vi "Parse multiple measurements to display - DLTS.vi"(0 "Array":T1[](array[typedef]) {"DLTS properties"."V range" items=["10mV"=0.01, "100mV"=0.1, "1V"=1.0, "10V"=10.0]; "DLTS properties"."I range" items=["10mV"=0.01, "100mV"=0.1, "1V"=1.0, "10V"=10.0]}, 5 "Session properties":T3, 7 "Workspace":path, 9 "Loop data":T4={"Persistent"={"Last file"=path "", "Last user"="", "Users"=[]}, "Temp handle"={"Connected"=FALSE, "Temp ctrl"={"Gain (P)"=0.0, "Reset (I)"=0.0, "Rate (D)"=0.0, "Stabilization rate"=0.0, "Stabilization delta"=0.0, "Type"=enum."Lake Shore 325", "Custom temp ctrl"={"VISA resource name"=""}, "Lakeshore 325"={"VISA name"="", "Loop"=0, "Heater Range"=1, "Heater Resistance"=0, "Sample sensor"=0, "Fast sensor"=0, "Slow sensor"=0}, "Lakeshore 331"={"VISA name"="", "Loop"=1, "Heater Range"=0, "Sample sensor"=0, "Fast sensor"=0, "Slow sensor"=0}, "Lakeshore 332"={"VISA name"="", "Loop"=1, "Heater Range"=0, "Sample sensor"=0, "Fast sensor"=0, "Slow sensor"=0}, "Lakeshore 335"={"VISA name"="", "Loop"=1, "Sample sensor"=0, "Fast sensor"=0, "Slow sensor"=0}}}, "Paths"={"Manual"=path "", "Settings"=path "", "Persistent"=path "", "Work dir."=path ""}, "Settings"={"MFIA"={"Address"="", "Use compensation"=TRUE, "Shut down gracefully"=FALSE}, "Temp ctrl"={"Gain (P)"=0.0, "Reset (I)"=0.0, "Rate (D)"=0.0, "Stabilization rate"=0.0, "Stabilization delta"=0.0, "Type"=enum."Lake Shore 325", "Custom temp ctrl"={"VISA resource name"=""}, "Lakeshore 325"={"VISA name"="", "Loop"=0, "Heater Range"=1, "Heater Resistance"=0, "Sample sensor"=0, "Fast sensor"=0, "Slow sensor"=0}, "Lakeshore 331"={"VISA name"="", "Loop"=1, "Heater Range"=0, "Sample sensor"=0, "Fast sensor"=0, "Slow sensor"=0}, "Lakeshore 332"={"VISA name"="", "Loop"=1, "Heater Range"=0, "Sample sensor"=0, "Fast sensor"=0, "Slow sensor"=0}, "Lakeshore 335"={"VISA name"="", "Loop"=1, "Sample sensor"=0, "Fast sensor"=0, "Slow sensor"=0}}, "Source-meter"={"Type"=enum."Custom", "Custom source-meter"={"VISA resource name"=""}, "Keithley 2600"={"VISA name"=""}}, "Other"={"Enable OriginLab"=FALSE, "Reader mode"=FALSE, "Auto-save"=FALSE}, "Defaults"={"IV properties"={"T"=0.0, "Vstart"=-0.5, "Vstop"=0.5, "Vpoints"=10.0, "Settling"=0.01, "I limit"=0.1, "Log mapping"=FALSE, "Averaging"=0.0}, "CV properties"={"T"=0.0, "Vstart"=-0.5, "Vstop"=0.5, "Vpoints"=10.0, "Precision"=enum."Normal", "Test signal"=0.01, "Auto I range"=FALSE, "Test frequency"=100000.0, "I range"=-2.0, "V range"=10.0, "Log mapping"=FALSE, "Rel perm"=0.0, "Area"=0.0}, "DLTS properties"={"Tstart"=0.0, "Instant start"=FALSE, "Tstop"=0.0, "T rate"=0.0, "Test signal"=0.0, "Test frequency"=0.0, "Bandwidth"=0.0, "Averaging"=0.0, "Vbias"=0.0, "Vpulse"=0.0, "pulse length"=0.0, "Pulse 2"=FALSE, "Vpulse 2"=0.0, "pulse length 2"=0.0, "I range"=-2.0, "V range"=10.0, "Emission rate"=[], "Sampling rate"=0.0, "Acq. delay"=0.0}, "LDLTS properties"={"T"=0.0, "Test signal"=0.0, "Test frequency"=0.0, "Bandwidth"=0.0, "Averaging"=0.0, "Vbias"=0.0, "Vpulse"=0.0, "pulse length"=0.0, "Pulse 2"=FALSE, "Vpulse 2"=0.0, "pulse length 2"=0.0, "I range"=-2.0, "V range"=10.0, "Sampling rate"=0.0, "Acq. delay"=0.0, "Sampling time"=0.0}}}, "Software version"=0.0, "MFIA handle"={"ziHandle"={"handleValid"=FALSE, "Conn"=0, "Path Prefix"="", "Handle"=0, "Connected"=FALSE, "Clockbase(s)"=0.0}, "Selected device"="", "ziModHandle"={"handleValid"=FALSE, "Conn"=0, "ModHandle"=0, "moduleID"="", "Path Prefix"=""}}, "Source-meter handle"={"Connected"=FALSE, "Source-meter"={"Type"=enum."Custom", "Custom source-meter"={"VISA resource name"=""}, "Keithley 2600"={"VISA name"=""}}}} {"MFIA handle"."ziModHandle"."ModHandle" format="0x%08x"; "MFIA handle"."ziModHandle"."Conn" format="0x%08x"; "MFIA handle"."ziHandle"."Handle" format="0x%08x"; "MFIA handle"."ziHandle"."Conn" format="0x%08x"; "Settings"."Defaults"."LDLTS properties"."V range" items=["10mV"=0.01, "100mV"=0.1, "1V"=1.0, "10V"=10.0]; "Settings"."Defaults"."LDLTS properties"."I range" items=["100nA"=-7.0, "1µA"=-6.0, "10µA"=-5.0, "100µA"=-4.0, "1mA"=-3.0, "10mA"=-2.0]; "Settings"."Defaults"."DLTS properties"."V range" items=["10mV"=0.01, "100mV"=0.1, "1V"=1.0, "10V"=10.0]; "Settings"."Defaults"."DLTS properties"."I range" items=["10mV"=0.01, "100mV"=0.1, "1V"=1.0, "10V"=10.0]; "Settings"."Defaults"."CV properties"."V range" items=["10mV"=0.01, "100mV"=0.1, "1V"=1.0, "10V"=10.0]; "Settings"."Defaults"."CV properties"."I range" items=["100nA"=-7.0, "1µA"=-6.0, "10µA"=-5.0, "100µA"=-4.0, "1mA"=-3.0, "10mA"=-2.0]; "Settings"."Defaults"."IV properties"."Settling" min=0.0 max=65535.0; "Settings"."Temp ctrl"."Lakeshore 335"."Slow sensor" items=["A", "B"]; "Settings"."Temp ctrl"."Lakeshore 335"."Fast sensor" items=["A", "B"]; "Settings"."Temp ctrl"."Lakeshore 335"."Sample sensor" items=["A", "B"]; "Settings"."Temp ctrl"."Lakeshore 335"."Loop" items=["Loop 1"=1, "Loop 2"=2]; "Settings"."Temp ctrl"."Lakeshore 332"."Slow sensor" items=["A", "B"]; "Settings"."Temp ctrl"."Lakeshore 332"."Fast sensor" items=["A", "B"]; "Settings"."Temp ctrl"."Lakeshore 332"."Sample sensor" items=["A", "B"]; "Settings"."Temp ctrl"."Lakeshore 332"."Heater Range" items=["Off", "Low (0.5W)", "Med (5W)", "High (50W)"]; "Settings"."Temp ctrl"."Lakeshore 332"."Loop" items=["Loop 1", "Loop 2"]; "Settings"."Temp ctrl"."Lakeshore 331"."Slow sensor" items=["A", "B"]; "Settings"."Temp ctrl"."Lakeshore 331"."Fast sensor" items=["A", "B"]; "Settings"."Temp ctrl"."Lakeshore 331"."Sample sensor" items=["A", "B"]; "Settings"."Temp ctrl"."Lakeshore 331"."Heater Range" items=["Off", "Low (0.5W)", "Med (5W)", "High (50W)"]; "Settings"."Temp ctrl"."Lakeshore 331"."Loop" items=["Loop 1", "Loop 2"]; "Settings"."Temp ctrl"."Lakeshore 325"."Slow sensor" items=["A", "B"]; "Settings"."Temp ctrl"."Lakeshore 325"."Fast sensor" items=["A", "B"]; "Settings"."Temp ctrl"."Lakeshore 325"."Sample sensor" items=["A", "B"]; "Settings"."Temp ctrl"."Lakeshore 325"."Heater Resistance" items=["25 Ohm"=1, "50 Ohm"=2]; "Settings"."Temp ctrl"."Lakeshore 325"."Heater Range" items=["Off", "Low (loop 1) or On (loop 2)", "High (loop 1)"]; "Settings"."Temp ctrl"."Lakeshore 325"."Loop" items=["Loop 1"=1, "Loop 2"=2]; "Temp handle"."Temp ctrl"."Lakeshore 335"."Slow sensor" items=["A", "B"]; "Temp handle"."Temp ctrl"."Lakeshore 335"."Fast sensor" items=["A", "B"]; "Temp handle"."Temp ctrl"."Lakeshore 335"."Sample sensor" items=["A", "B"]; "Temp handle"."Temp ctrl"."Lakeshore 335"."Loop" items=["Loop 1"=1, "Loop 2"=2]; "Temp handle"."Temp ctrl"."Lakeshore 332"."Slow sensor" items=["A", "B"]; "Temp handle"."Temp ctrl"."Lakeshore 332"."Fast sensor" items=["A", "B"]; "Temp handle"."Temp ctrl"."Lakeshore 332"."Sample sensor" items=["A", "B"]; "Temp handle"."Temp ctrl"."Lakeshore 332"."Heater Range" items=["Off", "Low (0.5W)", "Med (5W)", "High (50W)"]; "Temp handle"."Temp ctrl"."Lakeshore 332"."Loop" items=["Loop 1", "Loop 2"]; "Temp handle"."Temp ctrl"."Lakeshore 331"."Slow sensor" items=["A", "B"]; "Temp handle"."Temp ctrl"."Lakeshore 331"."Fast sensor" items=["A", "B"]; "Temp handle"."Temp ctrl"."Lakeshore 331"."Sample sensor" items=["A", "B"]; "Temp handle"."Temp ctrl"."Lakeshore 331"."Heater Range" items=["Off", "Low (0.5W)", "Med (5W)", "High (50W)"]; "Temp handle"."Temp ctrl"."Lakeshore 331"."Loop" items=["Loop 1", "Loop 2"]; "Temp handle"."Temp ctrl"."Lakeshore 325"."Slow sensor" items=["A", "B"]; "Temp handle"."Temp ctrl"."Lakeshore 325"."Fast sensor" items=["A", "B"]; "Temp handle"."Temp ctrl"."Lakeshore 325"."Sample sensor" items=["A", "B"]; "Temp handle"."Temp ctrl"."Lakeshore 325"."Heater Resistance" items=["25 Ohm"=1, "50 Ohm"=2]; "Temp handle"."Temp ctrl"."Lakeshore 325"."Heater Range" items=["Off", "Low (loop 1) or On (loop 2)", "High (loop 1)"]; "Temp handle"."Temp ctrl"."Lakeshore 325"."Loop" items=["Loop 1"=1, "Loop 2"=2]}, 11 "error in (no error)":errorcluster) -> (4 "Plot data":cluster{"2D data":dbl[], "2D data":dbl[]}[](array[cluster]), 6 "Plot names":string[](array[string]), 8 "X label":string, 10 "Y label":string, 15 "error out":errorcluster)   [LabVIEW 2019]
uses:
  Type defs/Loop data Type Def.ctl
  Type defs/Persistent Type Def.ctl
  Type defs/Temp handle Type Def.ctl
  Type defs/Temp ctrl Type Def.ctl
  Custom devices/Custom temp ctrl settings.ctl
  Type defs/Paths Type Def.ctl
  Type defs/Settings Type Def.ctl
  Type defs/Imps Type Def.ctl
  Type defs/Source-meter Type Def.ctl
  Custom devices/Custom source-meter settings.ctl
  Type defs/Other settings Type Def.ctl
  Type defs/IV properties Type Def.ctl
  Type defs/CV properties Type Def.ctl
  Type defs/DLTS properties Type Def.ctl
  Type defs/LDLTS properties Type Def.ctl
  Type defs/MFIA handle Type Def.ctl
  <instrlib>/Zurich Instruments LabOne/Public/ziTypeHandle.ctl
  <instrlib>/Zurich Instruments LabOne/Public/Modules/ziTypeModHandle.ctl
  Type defs/Source-meter handle Type Def.ctl
  Type defs/Session properties Type Def.ctl
  Type defs/cDLTS measurement Type Def.ctl
  <instrlib>/Zurich Instruments LabOne/Zurich Instruments LabOne.lvlib
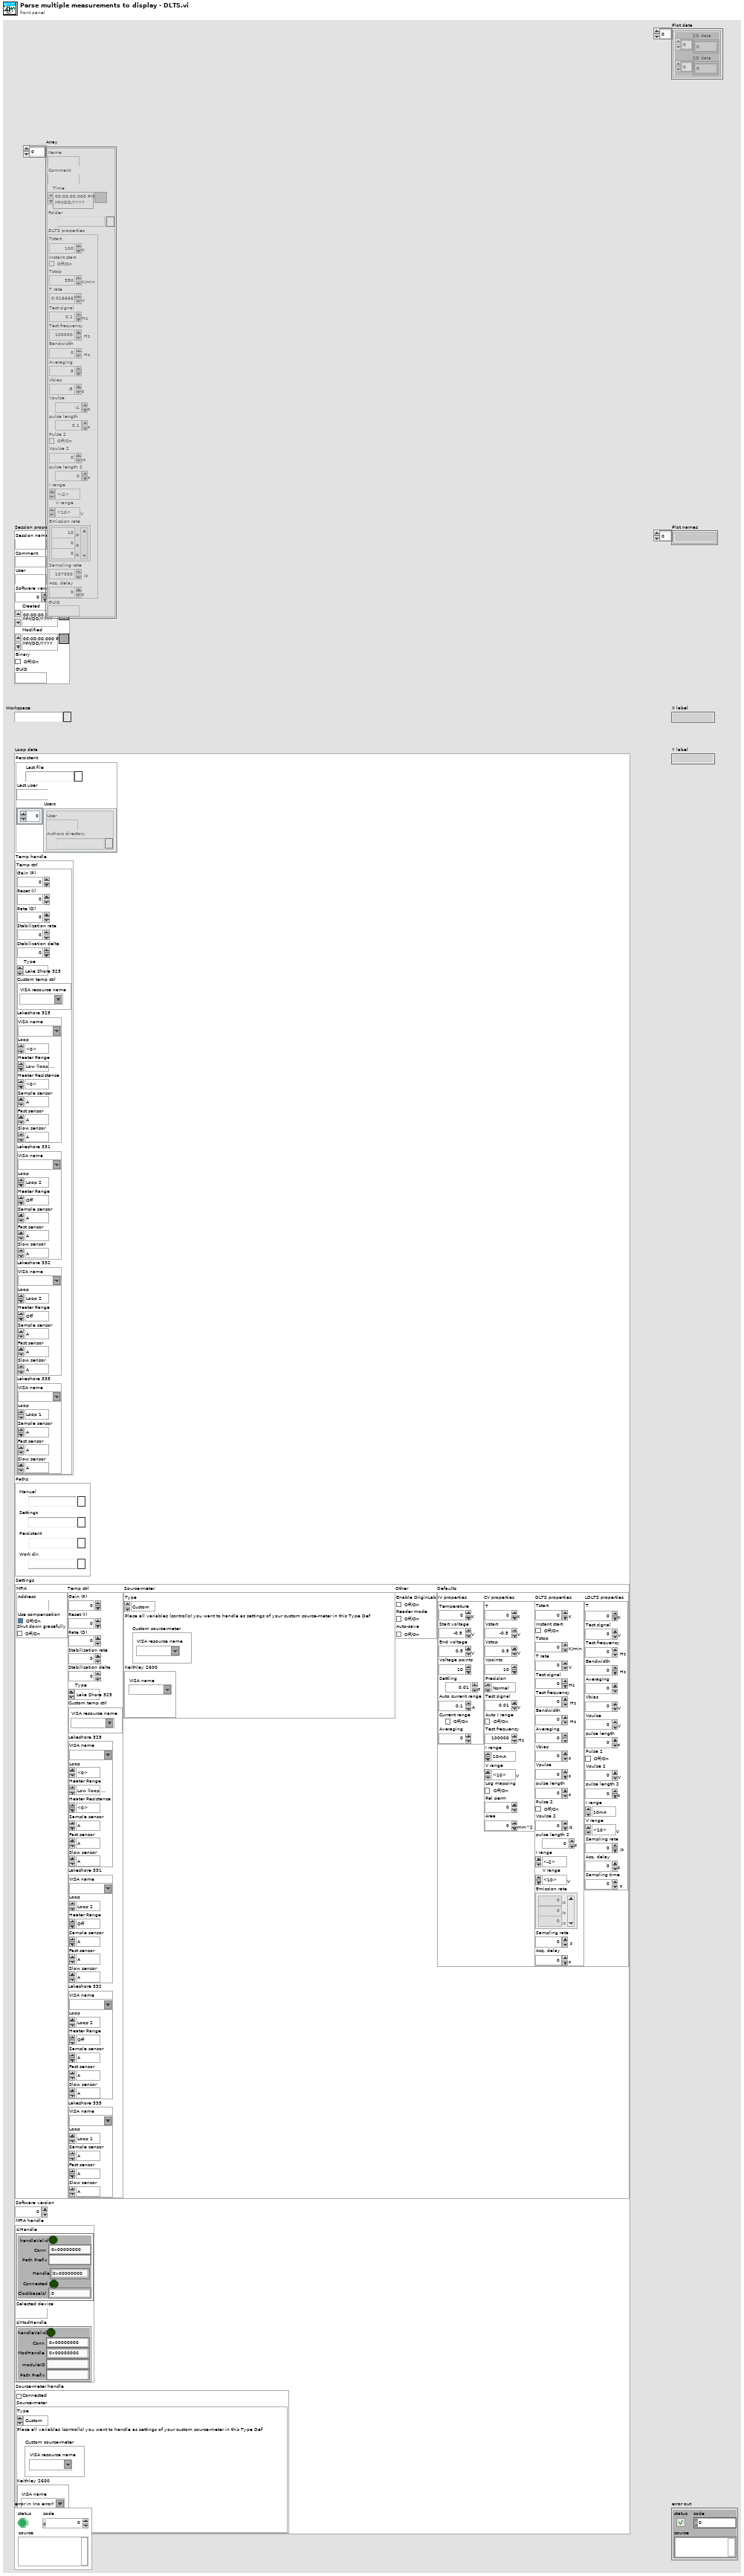
[diagram p1: front panel]
types:
  T1 = typedef "cDLTS measurement Type Def.ctl" = cluster{"Name":string, "Comment":string, "Time":timestamp, "Folder":path, "DLTS properties":T2, "GUID":string}
  T2 = typedef "DLTS properties Type Def.ctl" = cluster{"Tstart":dbl[unit], "Instant start":bool, "Tstop":dbl[unit], "T rate":dbl[unit], "Test signal":dbl[unit], "Test frequency":dbl[unit], "Bandwidth":dbl[unit], "Averaging":dbl, "Vbias":dbl[unit], "Vpulse":dbl[unit], "pulse length":dbl[unit], "Pulse 2":bool, "Vpulse 2":dbl[unit], "pulse length 2":dbl[unit], "I range":dbl, "V range":dbl[unit], "Emission rate":dbl[unit][], "Sampling rate":dbl[unit], "Acq. delay":dbl[unit]}
  T3 = typedef "Session properties Type Def.ctl" = cluster{"Session name":string, "Comment":string, "User":string, "Software version":dbl, "Created":timestamp, "Modified":timestamp, "Binary":bool, "GUID":string}
  T4 = typedef "Loop data Type Def.ctl" = cluster{"Persistent":T5, "Temp handle":T6, "Paths":T9, "Settings":T10, "Software version":dbl, "MFIA handle":T18, "Source-meter handle":T21}
  T5 = typedef "Persistent Type Def.ctl" = cluster{"Last file":path, "Last user":string, "Users":cluster{"User":string, "Authors directory":path}[]}
  T6 = typedef "Temp handle Type Def.ctl" = cluster{"Connected":bool, "Temp ctrl":T7}
  T7 = typedef "Temp ctrl Type Def.ctl" = cluster{"Gain (P)":dbl, "Reset (I)":dbl, "Rate (D)":dbl, "Stabilization rate":dbl, "Stabilization delta":dbl, "Type":enum16{"Custom", "Lake Shore 325", "Lake Shore 331", "Lake Shore 332", "Lake Shore 335"}, "Custom temp ctrl":T8, "Lakeshore 325":cluster{"VISA name":refnum<visa-resource-name>, "Loop":u16, "Heater Range":u16, "Heater Resistance":u16, "Sample sensor":u16, "Fast sensor":u16, "Slow sensor":u16}, "Lakeshore 331":cluster{"VISA name":refnum<visa-resource-name>, "Loop":u16, "Heater Range":u16, "Sample sensor":u16, "Fast sensor":u16, "Slow sensor":u16}, "Lakeshore 332":cluster{"VISA name":refnum<visa-resource-name>, "Loop":u16, "Heater Range":u16, "Sample sensor":u16, "Fast sensor":u16, "Slow sensor":u16}, "Lakeshore 335":cluster{"VISA name":refnum<visa-resource-name>, "Loop":u16, "Sample sensor":u16, "Fast sensor":u16, "Slow sensor":u16}}
  T8 = typedef "Custom temp ctrl settings.ctl" = cluster{"VISA resource name":refnum<visa-resource-name>}
  T9 = typedef "Paths Type Def.ctl" = cluster{"Manual":path, "Settings":path, "Persistent":path, "Work dir.":path}
  T10 = typedef "Settings Type Def.ctl" = cluster{"MFIA":T11, "Temp ctrl":T7, "Source-meter":T12, "Other":T14, "Defaults":cluster{"IV properties":T15, "CV properties":T16, "DLTS properties":T2, "LDLTS properties":T17}}
  T11 = typedef "Imps Type Def.ctl" = cluster{"Address":string, "Use compensation":bool, "Shut down gracefully":bool}
  T12 = typedef "Source-meter Type Def.ctl" = cluster{"Type":enum16{"Custom", "Keithley 2600"}, "Custom source-meter":T13, "Keithley 2600":cluster{"VISA name":refnum<visa-resource-name>}}
  T13 = typedef "Custom source-meter settings.ctl" = cluster{"VISA resource name":refnum<visa-resource-name>}
  T14 = typedef "Other settings Type Def.ctl" = cluster{"Enable OriginLab":bool, "Reader mode":bool, "Auto-save":bool}
  T15 = typedef "IV properties Type Def.ctl" = cluster{"T":dbl[unit], "Vstart":dbl[unit], "Vstop":dbl[unit], "Vpoints":dbl, "Settling":dbl[unit], "I limit":dbl[unit], "Log mapping":bool, "Averaging":dbl}
  T16 = typedef "CV properties Type Def.ctl" = cluster{"T":dbl[unit], "Vstart":dbl[unit], "Vstop":dbl[unit], "Vpoints":dbl, "Precision":enum16{"Low (Fast)", "Normal", "High (Slow)"}, "Test signal":dbl[unit], "Auto I range":bool, "Test frequency":dbl[unit], "I range":dbl, "V range":dbl[unit], "Log mapping":bool, "Rel perm":dbl, "Area":dbl[unit]}
  T17 = typedef "LDLTS properties Type Def.ctl" = cluster{"T":dbl[unit], "Test signal":dbl[unit], "Test frequency":dbl[unit], "Bandwidth":dbl[unit], "Averaging":dbl, "Vbias":dbl[unit], "Vpulse":dbl[unit], "pulse length":dbl[unit], "Pulse 2":bool, "Vpulse 2":dbl[unit], "pulse length 2":dbl[unit], "I range":dbl, "V range":dbl[unit], "Sampling rate":dbl[unit], "Acq. delay":dbl[unit], "Sampling time":dbl[unit]}
  T18 = typedef "MFIA handle Type Def.ctl" = cluster{"ziHandle":T19, "Selected device":string, "ziModHandle":T20}
  T19 = typedef "Zurich Instruments LabOne.lvlib/ziTypeHandle.ctl" = cluster{"handleValid":bool, "Conn":u64, "Path Prefix":string, "Handle":u64, "Connected":bool, "Clockbase(s)":dbl}
  T20 = typedef "Zurich Instruments LabOne.lvlib/ziTypeModHandle.ctl" = cluster{"handleValid":bool, "Conn":u64, "ModHandle":u64, "moduleID":string, "Path Prefix":string}
  T21 = typedef "Source-meter handle Type Def.ctl" = cluster{"Connected":bool, "Source-meter":T12}
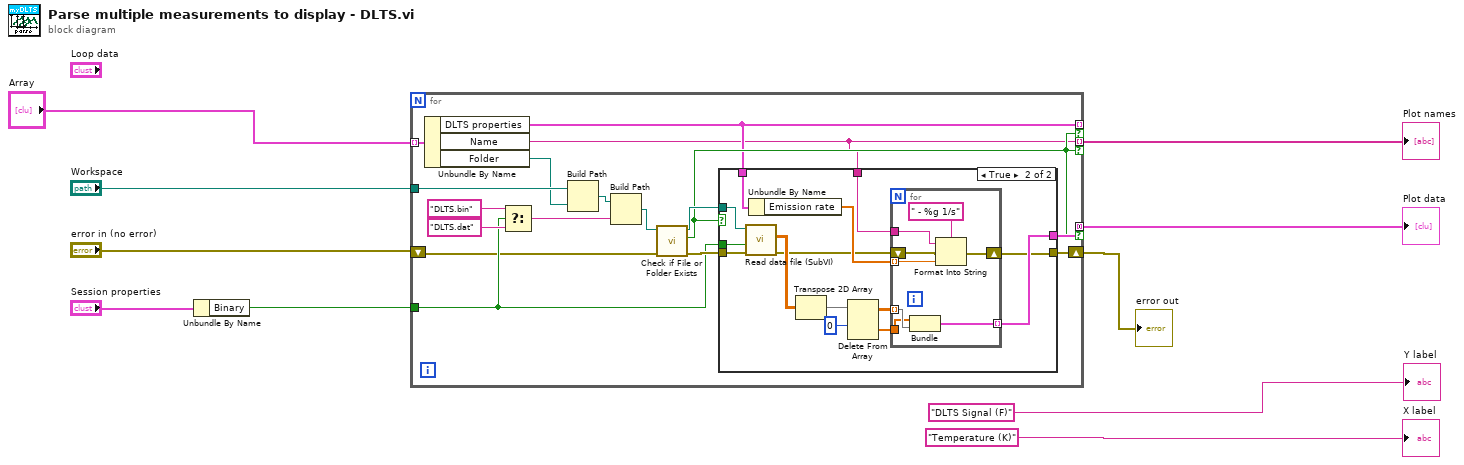
[diagram p0: block diagram]
diagram:
  n1 = Unbundle By Name("Session properties") -> ("Binary"=w3:bool)
  n2 = for {
    tunnel: w3 -> [w20]
    shift-right: [w18] -> w6
    shift-left: "error in (no error)" -> [w19]
    tunnel: [w17] -> w10 mode=concatenating if=w16
    tunnel: [w12] -> w9 mode=indexing if=w16
    tunnel: [w13] -> _ mode=indexing if=w16
    tunnel: "Workspace" -> [w15]
    tunnel: "Array" -> [w11] mode=indexing
    n3 = Unbundle By Name(w11) -> ("DLTS properties"=w13:T2, "Name"=w12:string, "Folder"=w14:path)
    n4 = Select(t="DLTS.bin", s=w20, f="DLTS.dat") -> (s? t:f=w23:string)
    n5 = Build Path(base path=w15, name or relative path=w14) -> (appended path=w27:path)
    n6 = Build Path(base path=w27, name or relative path=w23) -> (appended path=w26:path)
    n7 = call <vilib>:"Check if File or Folder Exists.vi"("error in (no error)"=w19, "path"=w26) -> ("error out"=w24:errorcluster, "file or folder exists?"=w16:bool, "dup path"=w25:path)  [unwired: 7 in]
    n8 = case shown="True" w16 {
      tunnel: w20 -> [_ w42]
      tunnel: w25 -> [_ w41]
      tunnel: w24 -> [w28 w40]
      tunnel: [w28 w30] -> w18
      tunnel: [_ w34] -> w17
      tunnel: w13 -> [_ w29]
      tunnel: w12 -> [_ w32]
      frame False {
      }
      frame True {
        n9 = call "Read data file (SubVI).vi"("error in"=w40, "Binary"=w42, "file path in"=w41) -> ("error out"=w31:errorcluster, "2D data"=w35:dbl[][])  [unwired: 6 in, 1 out]
        n10 = Unbundle By Name(w29) -> ("Emission rate"=w33:dbl[unit][])
        n11 = Transpose 2D Array(2D array=w35) -> (transposed array=w37:dbl[][])
        n12 = Delete From Array(array=w37, index (row)=0 ("disabled index (col)")) -> (deleted portion=w39:dbl[], array with subset deleted=w38:dbl[][])  [unwired: 2 in]
        n13 = for {
          tunnel: w38 -> [w50] mode=indexing
          tunnel: w39 -> [w49]
          tunnel: [w48] -> w34 mode=indexing
          tunnel: w33 -> [w46] mode=indexing
          tunnel: w32 -> [w47]
          shift-right: [w44] -> w30
          shift-left: w31 -> [w45]
          n14 = Bundle(w49, w50) -> (w48:cluster{dbl[], dbl[]})  [unwired: 1 in]
          n15 = Format Into String(format string=" - %g 1/s", initial string=w47, error in=w45, w46) -> (error out=w44:errorcluster)  [unwired: 1 out]
        }
      }
    }
  }
  "Plot data" <- w10
  "Plot names" <- w9
  "error out" <- w6
  "X label" <- "Temperature (K)"
  "Y label" <- "DLTS Signal (F)"
